vi "Enclose in Structure - Get Dummy Structure Reference.vi"(8 "error in":errorcluster, 11 "Structure Type":T1) -> (0 "error out":errorcluster, 3 "Structure Reference":refnum<vi>)   [LabVIEW 2020]
uses:
  <vilib>/platform/TimedLoop/XDataNode/XDataNode.xnode
  <vilib>/Platform/TimedLoop/XDataNode/nitl_modes.ctl
  <vilib>/Platform/TimedLoop/XDataNode/XDNodeRunTimeDep.lvlib
  <vilib>/Platform/TimedLoop/XDataNode/wakeup.ctl
  <vilib>/Platform/TimedLoop/XDataNode/timing_clust.ctl
  Enclose in Structure - Structure Type.ctl
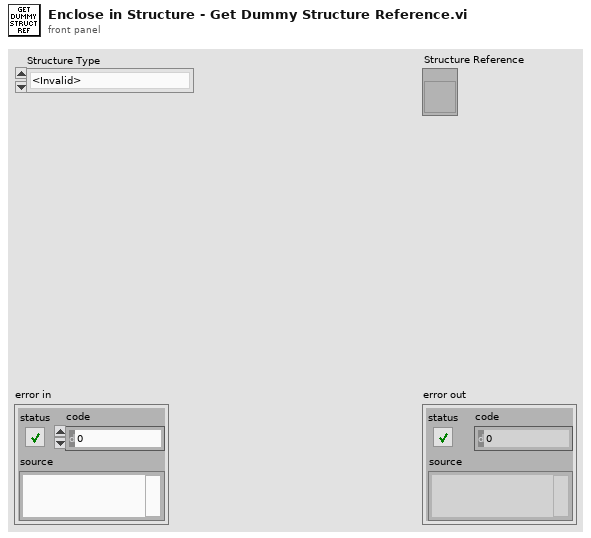
[diagram p1: front panel]
types:
  T1 = typedef "Enclose in Structure - Structure Type.ctl" = enum16{"<Invalid>", "For Loop", "While Loop", "Timed Loop", "Timed Sequence", "Case Structure", "Event Structure", "In Place Element Structure", "Flat Sequence", "Diagram Disable Structure", "Conditional Disable Structure", "Type Specialization Structure"}
  T2 = typedef "XDNodeRunTimeDep.lvlib/timing_clust.ctl" = cluster{"Expected End [f-1]":u64, "Actual End [f-1]":u64, "Finished Late? [f-1]":bool, "Expected End [i-1]":u64, "Actual End [i-1]":u64, "Finished Late? [i-1]":bool, "Expected Start [i]":u64, "Actual Start [i]":u64, "Expected Start [f]":u64, "Actual Start [f]":u64, "Source Name":string, "Structure Name":string, "Period":i64, "Deadline":i64, "Offset":i64, "Start":i64, "Priority":i32, "Timeout":i32, "Mode":T3, "Wakeup Reason":T4, "Error":errorcluster, "Source Type":string, "Secondary Source Type":string, "Global End Time":u64, "Global Start Time":u64, "Frame Duration":u64, "Iteration Duration":u64, "Assigned CPU":i32, "I/O Scan Engine Mode":u32}
  T3 = typedef "XDNodeRunTimeDep.lvlib/nitl_modes.ctl" = enum32{"No Change", "Process missed periods, maintain original phase", "Discard missed periods, maintain original phase", "Process missed periods, ignore original phase", "Discard missed periods, ignore original phase"}
  T4 = typedef "XDNodeRunTimeDep.lvlib/wakeup.ctl" = enum32{"Normal", "Aborted", "Asynchronous wakeup", "Timing source error", "Timed loop error", "Timeout"}
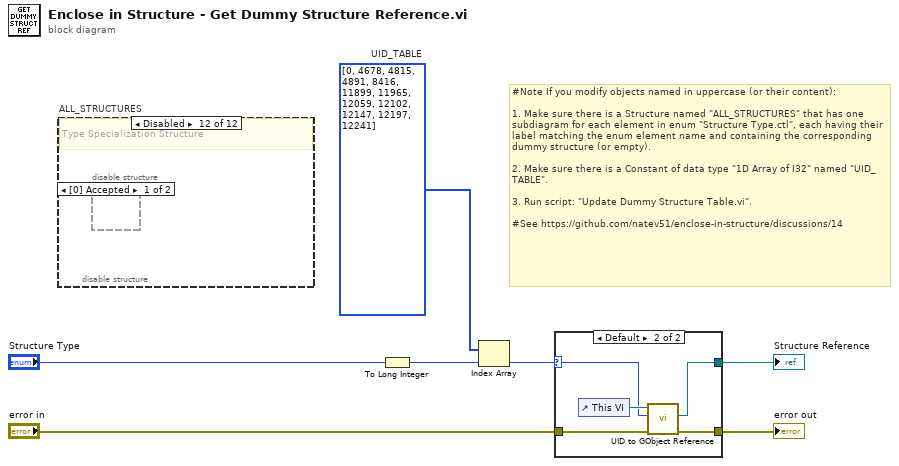
[diagram p0: block diagram]
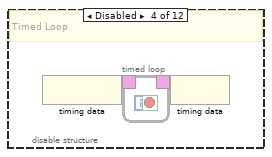
[diagram p6: hidden frame]
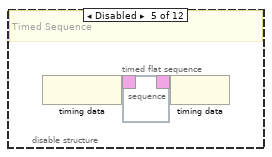
[diagram p7: hidden frame]
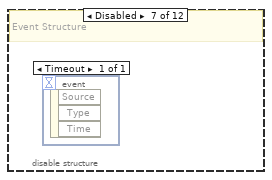
[diagram p10: hidden frame]
diagram:
  w6 = i32[] [0, 4678, 4815, 4891, 8416, 11899, 11965, 12059, 12102, 12147, 12197, 12241]  # UID_TABLE
  # "#Note If you modify objects named in uppercase (or their content):\n\n1. Make sure there is a Structure named \"ALL_STRUCTURES\" that has one subdiagram for each element in enum \"Structure Type.ctl\", each having their label matching the enum element name and containing the corresponding dummy structure (or empty).\n\n2. Make sure there is a Constant of data type \"1D Array of I32\" named \"UID_TABLE\".\n\n3. Run script: \"Update Dummy Structure Table.vi\".\n\n#See https://github.com/natev51/enclose-in-structure/discussions/14"
  n1 = disable-structure "ALL_STRUCTURES" shown="Disabled" {
    frame Enabled {
      # "<Invalid>"
    }
    frame Disabled {
      # "For Loop"
      n2 = for {
      }
    }
    frame Disabled {
      # "While Loop"
      n3 = while {
        stop <- _ stop-if-true
      }
    }
    frame Disabled {
      # "Timed Loop"
      n4 = node-c288() -> (w9:T2)
      n5 = timed-loop {
        timing: w9 -> [_]
        timing-out: [_] -> w8
        stop <- _ stop-if-true
      }
      n6 = node-c288(w8) -> ()
    }
    frame Disabled {
      # "Timed Sequence"
      n7 = node-c288() -> (w15:T2)
      n8 = timed-sequence {
        timing: w15 -> [_]
        timing-out: [_] -> w14
        n9 = timed-flat-sequence {
        }
      }
      n10 = node-c288(w14) -> ()
    }
    frame Disabled {
      # "Case Structure"
      n11 = case shown="False" {
        selector: _ -> [_ _]
        frame False {
        }
        frame True {
        }
      }
    }
    frame Disabled {
      # "Event Structure"
      n12 = event shown="[0] Timeout" {
        selector: _ -> [_]
        dyn-events: _ -> [_]
        timeout: _ -> [_]
        event Timeout {
          n13 = event-data() -> ()  [unwired: 1 in, 3 out]
        }
      }
    }
    frame Disabled {
      # "In Place Element Structure"
      n14 = in-place {
      }
    }
    frame Disabled {
      # "Flat Sequence"
      n15 = flat-sequence {
        frame #0 {
        }
      }
    }
    frame Disabled {
      # "Diagram Disable Structure"
      n16 = disable-structure shown="Disabled" {
        frame Disabled {
        }
        frame Enabled {
        }
      }
    }
    frame Disabled {
      # "Conditional Disable Structure"
      n17 = disable-structure shown="Default" {
        frame Enabled {
        }
      }
    }
    frame Disabled {
      # "Type Specialization Structure"
      n18 = disable-structure shown="[0] Accepted" {
        frame Enabled {
        }
        frame Disabled {
        }
      }
    }
  }
  n19 = To Long Integer(number="Structure Type") -> (32bit integer=w3:i32)
  n20 = Index Array(array=w6, index=w3) -> (element=w5:i32)
  n21 = case shown="Default" w5 {
    selector: w5 -> [_ w23]
    tunnel: "error in" -> [w20 w25]
    tunnel: [w20 w22] -> w2
    tunnel: [_ w21] -> w1
    frame ..0 {
    }
    frame Default {
      n22 = control-ref of="This VI"() -> (w24:refnum<vi>)
      n23 = call <vilib>:"UID to GObject Reference.vi"("error in (no error)"=w25, "UID"=w23, "Owning VI"=w24) -> ("error out"=w22:errorcluster, "GObject"=w21:refnum<vi>)  [unwired: 6 in, 1 out]
    }
  }
  "error out" <- w2
  "Structure Reference" <- w1
